vi "niRFUtil WFM Apply Linear Gain (complex WDT).vi"(1 "Gain":sgl=1.0 format="%.2f", 3 "Real WDT In":T1) -> (0 "Real WDT Out":T1)   [LabVIEW 2015, in "niRFUtil.lvlib"]
doc: "(c) Copyright 2006, National Instruments, Inc. This VI may not be duplicated, sold, or distributed without written consent from National Instruments."
uses:
  niRFUtil.lvlib
  Includes/niRFUtil INC Real WDT.ctl
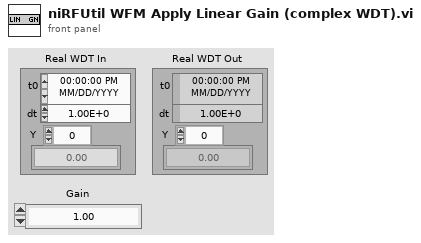
[diagram p1: front panel]
types:
  T1 = typedef "niRFUtil.lvlib/niRFUtil INC Real WDT.ctl" = waveform(sgl)
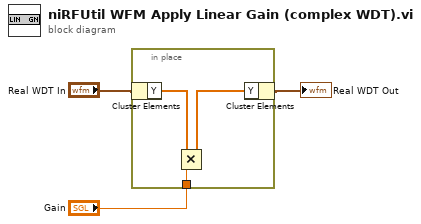
[diagram p0: block diagram]
diagram:
  n1 = in-place {
    in-place-border: "Gain" -> [w6]
    n2 = in-place-cluster #1("Real WDT In") -> ("Y"=w5:sgl[])
    n3 = Multiply(x=w5, y=w6) -> (x*y=w4:sgl[])
    n4 = in-place-cluster #1("Y"=w4) -> (→"Real WDT Out":T1)
  }
